vi "LoadTestSteps.vi"(8 "error in (no error)":errorcluster, 11 "TestSeqClass in":refnum<class "TestSeqClass.lvclass">) -> (0 "error out":errorcluster, 3 "TestSeqClass out":refnum<class "TestSeqClass.lvclass">)   [LabVIEW 2019, in "TestSeqClass.lvclass"]
doc: "Scancon A/S"
uses:
  TestSeqClass.lvclass
  TestSeqClass.lvclass/TestSeqClass.ctl
  GUIHandler_Main/GUI_Handler_Main.lvclass
  TestMeasureStep/TestMeasureStep.lvclass
  GUIHandler/GUI_Handler_Seq.lvclass
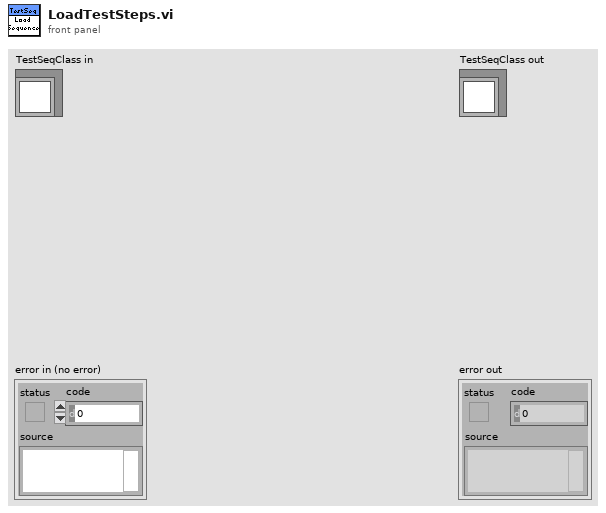
[diagram p1: front panel]
types:
  T1 = enum16{"open", "open or create", "create or replace", "create", "open (read only)"}
  T2 = typedef "TestTypeSelect.ctl" = enum16{"Calibration", "Testing"}
  T3 = typedef "TestSeqType.ctl" = refnum<class "TestMeasureStep.lvclass">[]
  T4 = typedef "TestSeqClass.lvclass/TesstepType.ctl" = cluster{"TestName":string, "Meas":dbl, "Min ":dbl, "Max":dbl, "TestStatus":T5, "StringLimit":string, "StringMeas":string, "Unit":string}
  T5 = typedef "TestStatus.ctl" = enum16{"Not Executed", "Passed", "Failed", "Inconclusive", "Processing"}
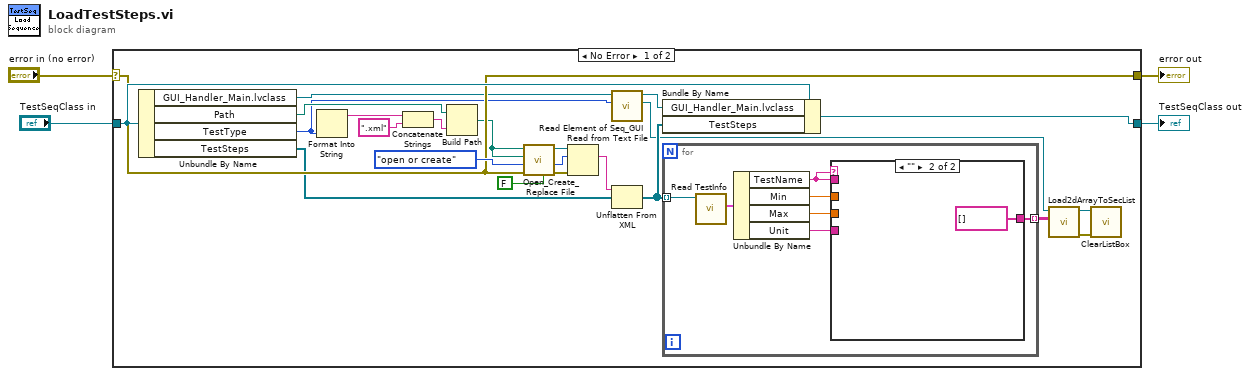
[diagram p0: block diagram]
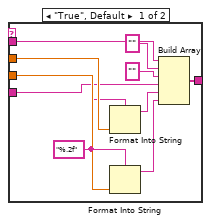
[diagram p2: hidden frame]
diagram:
  n1 = case shown="No Error" "error in (no error)" {
    selector: "error in (no error)" -> [w17 w47]
    tunnel: [w17 w47] -> w3
    tunnel: [w27 w46] -> w1
    tunnel: "TestSeqClass in" -> [w21 w46]
    frame No Error {
      n2 = Unbundle By Name(w21) -> ("GUI_Handler_Main.lvclass"=w10:refnum<class "GUI_Handler_Main.lvclass">, "Path"=w20:path, "TestType"=w7:T2, "TestSteps"=w16:T3)
      n3 = Format Into String(w7) -> (resulting string=w11:string)  [unwired: 3 in, 1 out]
      n4 = Concatenate Strings(w11, ".xml" ("string")) -> (w19:string)
      n5 = Build Path(base path=w20, name or relative path=w19) -> (appended path=w13:path)
      n6 = call <vilib>:"Open_Create_Replace File.vi"("advisory dialog? (display:T)"=FALSE, "error in (no error)"=w17, "function (open:0)"=T1."open or create", "start path  (Not A Path)"=w13, "file path"=w13) -> ("error out"=w25:errorcluster, "file size (bytes)"=w23:i32, "refnum"=w24:refnum<file>)  [unwired: 2 in, 2 out]
      n7 = Read from Text File(file (use dialog)=w24, count=w23, error in=w25) -> (text=w22:string)  [unwired: 1 in, 3 out]
      n8 = call-dynamic "Read Element of Seq_GUI.vi"("Variant"=w7, "GUI_Handler_Main in"=w10) -> ("GUI_Handler_Seq.lvclass"=w9:refnum<class "GUI_Handler_Seq.lvclass">, "GUI_Handler_Main out"=w8:refnum<class "GUI_Handler_Main.lvclass">)  [unwired: 7 in, 1 out]
      n9 = Unflatten From XML(xml string=w22, type=w16) -> (value=w15:T3)  [unwired: 1 in, 1 out]
      n10 = Bundle By Name(cluster=w21, "GUI_Handler_Main.lvclass"=w8, "TestSteps"=w15) -> (w27:refnum<class "TestSeqClass.lvclass">)
      n11 = for {
        tunnel: w15 -> [w30] mode=indexing
        tunnel: [w32] -> w12 mode=indexing
        n12 = call-dynamic "Read TestInfo.vi"("TestMeasureStep in"=w30) -> ("TestInfo 2"=w29:T4)  [unwired: 8 in, 2 out]
        n13 = Unbundle By Name(w29) -> ("TestName"=w28:string, "Min"=w34:dbl, "Max"=w33:dbl, "Unit"=w31:string)
        n14 = case shown="\"\"" w28 {
          tunnel: w28 -> [w44 _]
          tunnel: w34 -> [w42 _]
          tunnel: w33 -> [w41 _]
          tunnel: [w39 string[] []] -> w32
          tunnel: w31 -> [w37 _]
          frame "True", Default {
            w40 = "%.2f" ("format string")
            n15 = Format Into String(format string=w40, w42) -> (resulting string=w36:string)  [unwired: 2 in, 1 out]
            n16 = Format Into String(format string=w40, w41) -> (resulting string=w35:string)  [unwired: 2 in, 1 out]
            n17 = Build Array(w44, "" ("element"), "" ("element"), w37, w36, w35) -> (w39:string[])
          }
          frame "" {
          }
        }
      }
      n18 = call-dynamic "Load2dArrayToSecList.vi"("Item Names"=w12, "GUI_Handler in"=w9) -> ("error out"=w5:errorcluster, "GUI_Handler out"=w6:refnum<class "GUI_Handler_Seq.lvclass">)  [unwired: 8 in]
      n19 = call-dynamic "ClearListBox.vi"("error in (no error)"=w5, "GUI_Handler_Seq in"=w6) -> ()  [unwired: 8 in, 2 out]
    }
    frame Error {
    }
  }
  "error out" <- w3
  "TestSeqClass out" <- w1
